vi "Append Flattened Pixmap to Report.vi"(4 "MS Office parameters":T1, 6 "caption or alt string":string, 7 "alignment (default)":T3, 8 "error in (no error)":errorcluster, 9 "image data":T2, 10 "image format (jpeg)":enum32{"PNG", "JPEG", "GIF"}(ring), 11 "report in":refnum<class "NI_report.lvclass">) -> (0 "error out":errorcluster, 1 "end out (word)":i32, 2 "start out (word)":i32, 3 "report out":refnum<class "NI_report.lvclass">)   [LabVIEW 2020, in "NI_ReportGenerationCore.lvlib"]
uses:
  <vilib>/Utility/NIReport.llb/NI_ReportGenerationCore.lvlib
  <vilib>/Utility/NIReport.llb/HTML Report Image Alignment.ctl
  <vilib>/Utility/NIReport.llb/NI_report.lvclass
  <vilib>/picture/picture.llb/imagedata.ctl
  <vilib>/printing/ReportDocExtensions.llb/File_types_for_reports.ctl
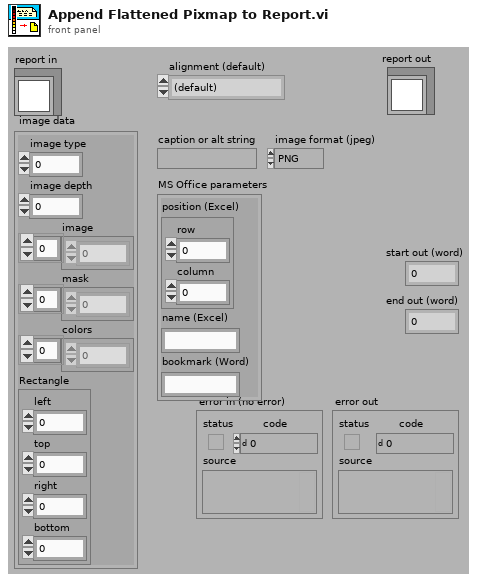
[diagram p1: front panel]
types:
  T1 = cluster{"position (Excel)":cluster{"row":i32, "column":i32}, "name (Excel)":string, "bookmark (Word)":string}
  T2 = typedef "imagedata.ctl" = cluster{"image type":i32, "image depth":i32, "image":u8[], "mask":u8[], "colors":u32[], "Rectangle":cluster{"left":i16, "top":i16, "right":i16, "bottom":i16}}
  T3 = typedef "NI_ReportGenerationCore.lvlib/HTML Report Image Alignment.ctl" = enum16{"(default)", "LEFT", "RIGHT", "TOP", "TEXTTOP", "MIDDLE", "ABSMIDDLE", "BASELINE", "BOTTOM", "ABSBOTTOM"}
  T4 = typedef "NI_ReportGenerationCore.lvlib/File_types_for_reports.ctl" = enum16{".jpg", ".png", ".html", ".gif"}
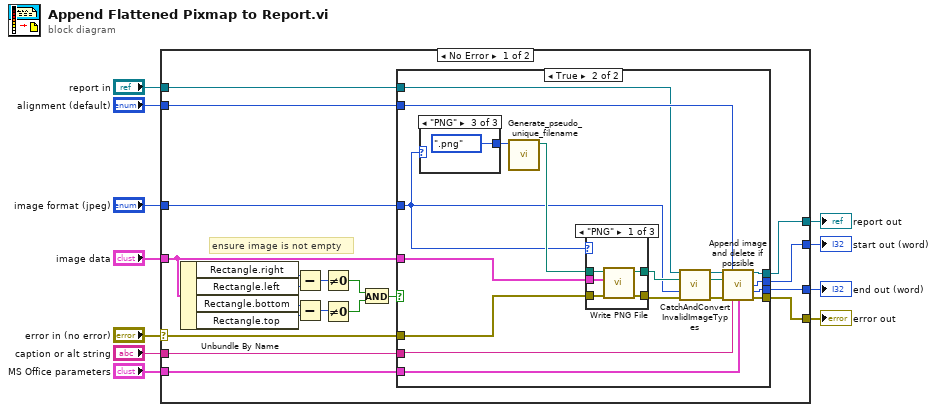
[diagram p0: block diagram]
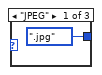
[diagram p3: hidden frame]
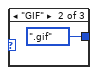
[diagram p4: hidden frame]
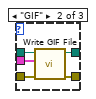
[diagram p5: hidden frame]
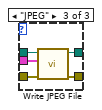
[diagram p6: hidden frame]
diagram:
  n1 = case shown="No Error" "error in (no error)" {
    selector: "error in (no error)" -> [w12 w70]
    tunnel: "caption or alt string" -> [w31 _]
    tunnel: "alignment (default)" -> [w30 _]
    tunnel: [w29 w71] -> w9
    tunnel: "report in" -> [w28 w71]
    tunnel: [w27 w70] -> w7
    tunnel: "image format (jpeg)" -> [w26 _]
    tunnel: "image data" -> [w25 _]
    tunnel: [w15 _] -> w4
    tunnel: [w14 _] -> w3
    tunnel: "MS Office parameters" -> [w13 _]
    frame No Error {
      # "ensure image is not empty"
      n2 = Unbundle By Name(w25) -> ("Rectangle.right"=w23:i16, "Rectangle.left"=w24:i16, "Rectangle.bottom"=w22:i16, "Rectangle.top"=w21:i16)
      n3 = Subtract(x=w23, y=w24) -> (x-y=w19:i16)
      n4 = Subtract(x=w22, y=w21) -> (x-y=w20:i16)
      n5 = Not Equal To 0?(x=w19) -> (x != 0?=w18:bool)
      n6 = Not Equal To 0?(x=w20) -> (x != 0?=w17:bool)
      n7 = And(x=w18, y=w17) -> (x .and. y?=w16:bool)
      n8 = case shown="True" w16 {
        tunnel: w12 -> [w32 w51]
        tunnel: w31 -> [_ w50]
        tunnel: w30 -> [_ w49]
        tunnel: [w33 w48] -> w29
        tunnel: w28 -> [w33 w46]
        tunnel: [w32 w43] -> w27
        tunnel: w26 -> [_ w38]
        tunnel: w25 -> [_ w37]
        tunnel: [_ w35] -> w15
        tunnel: [_ w34] -> w14
        tunnel: w13 -> [_ w36]
        frame False {
        }
        frame True {
          n9 = case shown="\"PNG\"" w38 {
            tunnel: [File_types_for_reports.".jpg" ("file type(.jpg)") File_types_for_reports.".gif" ("file type(.jpg)") File_types_for_reports.".png" ("file type(.jpg)")] -> w40
            frame "JPEG" {
            }
            frame "GIF" {
            }
            frame "PNG" {
            }
          }
          n10 = call <vilib>:"Generate_pseudo_unique_filename.vi"("file type(.jpg)"=w40) -> ("generated path"=w39:path)  [unwired: 8 in, 2 out]
          n11 = case shown="\"PNG\"" w38 {
            tunnel: w51 -> [w57 w64 w67]
            tunnel: [w56 w63 w65] -> w41
            tunnel: [w55 w60 w66] -> w47
            tunnel: w39 -> [w59 w62 w69]
            tunnel: w37 -> [w58 w61 w68]
            frame "PNG" {
              n12 = call <vilib>:"Write PNG File.vi"("error in (no error)"=w57, "image data"=w58, "path to PNG file"=w59) -> ("error out"=w56:errorcluster, "path"=w55:path)  [unwired: 7 in]
            }
            frame "GIF" {
              n13 = call <vilib>:"Write GIF File.vi"("error in (no error)"=w64, "image data"=w61, "path to GIF file"=w62) -> ("error out"=w63:errorcluster, "path"=w60:path)  [unwired: 7 in]
            }
            frame "JPEG" {
              n14 = call <vilib>:"Write JPEG File.vi"("error in (no error)"=w67, "image data"=w68, "path to JPEG file"=w69) -> ("error out"=w65:errorcluster, "path"=w66:path)  [unwired: 7 in]
            }
          }
          n15 = call-dynamic "CatchAndConvertInvalidImageTypes.vi"("report in"=w46, "path to image"=w47, "image format (jpeg)"=w38, "error in (no error)"=w41) -> ("report out"=w45:refnum<class "NI_report.lvclass">, "path to image out"=w44:path, "error out"=w42:errorcluster)  [unwired: 9 in]
          n16 = call-dynamic "Append image and delete if possible.vi"("report in"=w45, "alignment (default)"=w49, "path to image"=w44, "error in (no error)"=w42, "caption or alternative string"=w50, "MS Office parameters"=w36) -> ("report out"=w48:refnum<class "NI_report.lvclass">, "start out Word)"=w35:i32, "end out Word)"=w34:i32, "error out"=w43:errorcluster)  [unwired: 6 in]
        }
      }
    }
    frame Error {
    }
  }
  "report out" <- w9
  "error out" <- w7
  "start out (word)" <- w4
  "end out (word)" <- w3
